vi "State_Machine.vi"(8 "error in (no error)":errorcluster caption="entrée d'erreur (pas d'erreur)", 11 "Get_Voltage en entrée":refnum<class "Nodon_Set_State_RS.lvclass">) -> (0 "error out":errorcluster caption="sortie d'erreur", 2 "Json_String":string, 3 "Get_Voltage en sortie":refnum<class "Nodon_Set_State_RS.lvclass">)   [LabVIEW 2020, in "Library Test.lvlib" / "Nodon_Set_State_RS.lvclass"]
uses:
  Nodon_Set_State_RS.lvclass
  C:/Users/ngarcin/OneDrive - Altyor/Standard TB/Class/Test/Test (Default)/Test (Default).lvclass
  C:/Users/ngarcin/OneDrive - Altyor/Standard TB/Class/Test/Nodon_Send_Command_UART/Nodon_Send_Command_UART.lvclass
  JSON API/JSON Value/Set from JSON string.vi
  JSON API/JSON Value/JSON Value.lvclass
  Nodon_Send_Command_UART.lvclass
  Nodon_Set_State_RS.lvclass/Nodon_Set_State_RS.ctl
  JSON API/Variant JSON/Variant JSON.lvlib
  JSON API/Get Polymorphic/JSON GetSet.lvlib
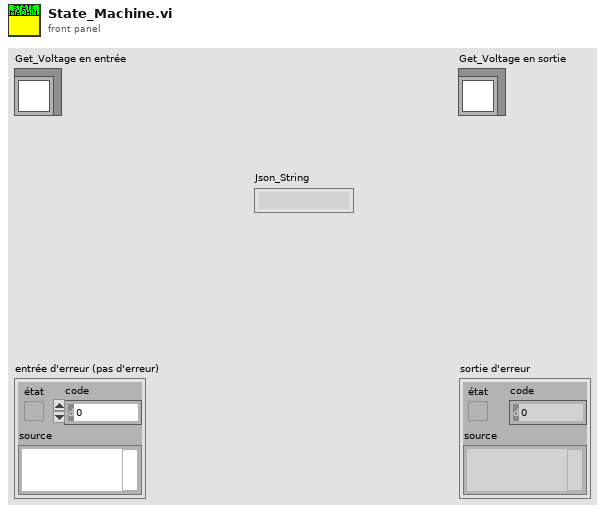
[diagram p1: front panel]
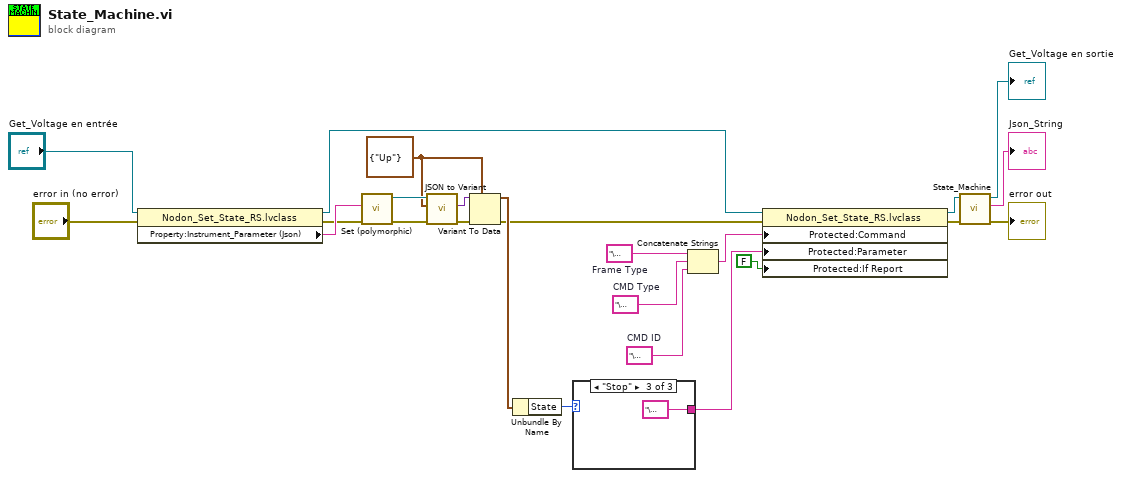
[diagram p0: block diagram]
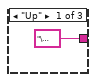
[diagram p2: hidden frame]
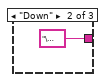
[diagram p3: hidden frame]
diagram:
  w8 = cluster{"State":enum16{"Up", "Down", "Stop"}} {"State"=enum."Up"}
  w19 = "\u0000"  # Frame Type
  w18 = "\u0010"  # CMD ID
  w17 = "\u0000"  # CMD Type
  n1 = property class="Nodon_Set_State_RS.lvclass"(reference="Get_Voltage en entrée", error in="error in (no error)") -> (reference out=w5:refnum<class "Nodon_Set_State_RS.lvclass">, error out=w10:errorcluster, "Property:Instrument_Parameter (Json)"=w11:string)
  n2 = call-poly "Set (polymorphic).vi"("error in (no error)"=w10, "JSON stream"=w11) -> ("error out"=w13:errorcluster, "JSON Value out"=w15:refnum<class "JSON Value.lvclass">)  [unwired: 7 in, 1 out]
  n3 = call "JSON to Variant.vi"("error in (no error)"=w13, "Variant (Data Type)"=w8, "JSON Value"=w15) -> ("error out"=w14:errorcluster, "Variant out"=w12:variant)  [unwired: 7 in]
  n4 = Variant To Data(error in=w14, type=w8, Variant=w12) -> (data=w7:cluster{"State":enum16{"Up", "Down", "Stop"}}, error out=w3:errorcluster)
  n5 = Unbundle By Name(w7) -> ("State"=w2:enum16{"Up", "Down", "Stop"})
  n6 = case shown="\"Stop\"" w2 {
    tunnel: ["\u0001" ("Chaîne") "\u0002" ("Chaîne") "\u0003" ("Chaîne")] -> w1
    frame "Up" {
    }
    frame "Down" {
    }
    frame "Stop" {
    }
  }
  n7 = Concatenate Strings(w19, w17, w18) -> (w16:string)
  n8 = property class="Nodon_Set_State_RS.lvclass"(reference=w5, error in=w3, "Protected:Command"=w16, "Protected:Parameter"=w1, "Protected:If Report"=FALSE ("If Report")) -> (reference out=w21:refnum<class "Nodon_Set_State_RS.lvclass">, error out=w20:errorcluster)
  n9 = call-parent "State_Machine.vi"("error in (no error)"=w20, "Send_Frame en entrée"=w21) -> ("error out"=→"error out":errorcluster, "Json_String"=→"Json_String":string, "Send_Frame en sortie"=→"Get_Voltage en sortie":refnum<class "Nodon_Set_State_RS.lvclass">)  [unwired: 7 in]
